vi "OculusRift INTERFACE VI.vi"() -> ()   [LabVIEW 2014]
uses:
  <vilib>/Platform/TimedLoop/XDataNode/timing_clust.ctl
  <vilib>/Platform/TimedLoop/XDataNode/nitl_modes.ctl
  <vilib>/Platform/TimedLoop/XDataNode/wakeup.ctl
  <vilib>/Platform/TimedLoop/XDataNode/XDataNode.xnode
  <vilib>/Platform/TimedLoop/XDataNode/XDNodeRunTimeDep.lvlib
panel:
  in  "LOOP CS":i64=200
  in  "LOOP OR":i64
  in  "service name":string="localhost"
  in  "port":u16=6340
  out "error out":errorcluster
  out "data out":string
  in  "error in (no error) 2":errorcluster
  in  "error in (no error)":errorcluster
  in  "OR Port":u16=52717
  in  "Oculus Rift Adress":string="localhost"
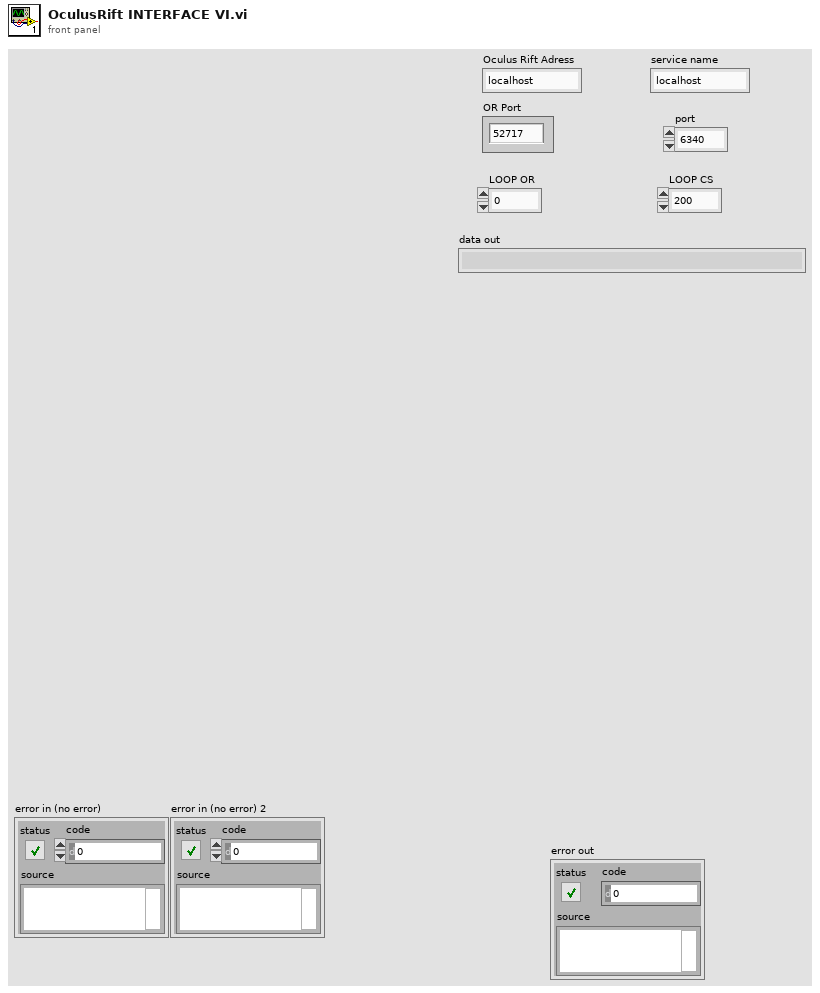
[diagram p1: front panel]
types:
  T1 = typedef "XDNodeRunTimeDep.lvlib/timing_clust.ctl" = cluster{"Expected End [f-1]":u64, "Actual End [f-1]":u64, "Finished Late? [f-1]":bool, "Expected End [i-1]":u64, "Actual End [i-1]":u64, "Finished Late? [i-1]":bool, "Expected Start [i]":u64, "Actual Start [i]":u64, "Expected Start [f]":u64, "Actual Start [f]":u64, "Source Name":string, "Structure Name":string, "Period":i64, "Deadline":i64, "Offset":i64, "Start":i64, "Priority":i32, "Timeout":i32, "Mode":T2, "Wakeup Reason":T3, "Error":errorcluster, "Source Type":string, "Secondary Source Type":string, "Global End Time":u64, "Global Start Time":u64, "Frame Duration":u64, "Iteration Duration":u64, "Assigned CPU":i32, "I/O Scan Engine Mode":u32}
  T2 = typedef "XDNodeRunTimeDep.lvlib/nitl_modes.ctl" = enum32{"No Change", "Process missed periods, maintain original phase", "Discard missed periods, maintain original phase", "Process missed periods, ignore original phase", "Discard missed periods, ignore original phase"}
  T3 = typedef "XDNodeRunTimeDep.lvlib/wakeup.ctl" = enum32{"Normal", "Aborted", "Asynchronous wakeup", "Timing source error", "Timed loop error", "Timeout"}
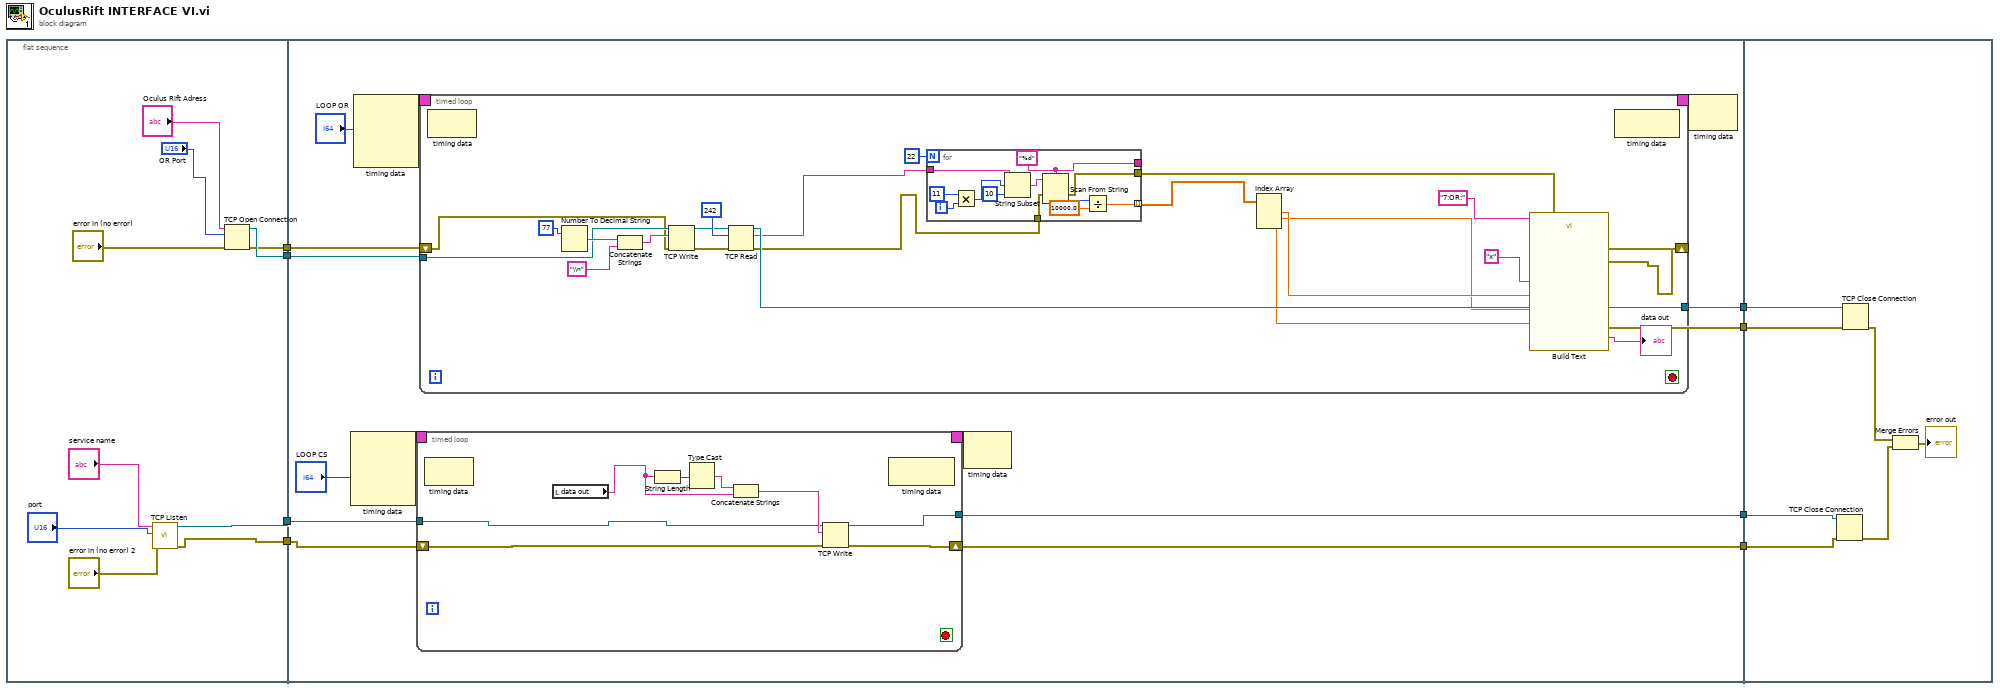
[diagram p0: block diagram]
diagram:
  n1 = flat-sequence {
    tunnel: [w18] -> w8
    tunnel: [w17] -> w7
    tunnel: [w14] -> w6
    tunnel: [w15] -> w1
    tunnel: w8 -> [w30]
    tunnel: w7 -> [w29]
    tunnel: w6 -> [w28]
    tunnel: [w27] -> w5
    tunnel: [w26] -> w4
    tunnel: [w25] -> w3
    tunnel: [w24] -> w2
    tunnel: w1 -> [w22]
    tunnel: w5 -> [w92]
    tunnel: w4 -> [w91]
    tunnel: w3 -> [w90]
    tunnel: w2 -> [w89]
    frame #0 {
      n2 = call <vilib>:"TCP Listen.vi"("error in (no error)"="error in (no error) 2", "port"="port", "service name"="service name") -> ("error out"=w14:errorcluster, "connection ID"=w15:refnum<k5>)  [unwired: 4 in, 3 out]
      n3 = TCP Open Connection(address="Oculus Rift Adress", remote port or service name="OR Port", error in (no error)="error in (no error)") -> (connection ID=w18:refnum<k5>, error out=w17:errorcluster)  [unwired: 2 in]
    }
    frame #1 {
      n4 = node-c288("LOOP CS") -> (w32:T1)  [unwired: 3 in]
      n5 = node-c288("LOOP OR") -> (w21:T1)  [unwired: 3 in]
      n6 = timed-loop {
        timing: w32 -> [_]
        timing-out: [_] -> w31
        shift-right: [w79] -> w26
        shift-left: w28 -> [w73]
        tunnel: [w78] -> w27
        tunnel: w22 -> [w74]
        stop <- _ stop-if-true
        n7 = node-c288() -> ()  [unwired: 1 in, 1 out]
        n8 = local read "data out"() -> (w72:string)
        n9 = String Length(string=w72) -> (length=w77:i32)
        n10 = Type Cast(x=w77) -> (*(type *) &x=w76:string)  [unwired: 1 in]
        n11 = Concatenate Strings(w76, w72) -> (w75:string)
        n12 = TCP Write(connection ID=w74, data in=w75, error in (no error)=w73) -> (connection ID out=w78:refnum<k5>, error out=w79:errorcluster)  [unwired: 1 in, 1 out]
        n13 = node-c288() -> ()  [unwired: 1 in, 1 out]
      }
      n14 = timed-loop {
        timing: w21 -> [_]
        timing-out: [_] -> w20
        tunnel: w30 -> [w46]
        shift-right: [w34] -> w24
        shift-left: w29 -> [w45]
        tunnel: [w44] -> w25
        stop <- _ stop-if-true
        n15 = node-c288() -> ()  [unwired: 1 in, 1 out]
        n16 = Number To Decimal String(number=77) -> (decimal integer string=w49:string)  [unwired: 1 in]
        n17 = Concatenate Strings(w49, "\\n" ("string")) -> (w47:string)
        n18 = TCP Write(connection ID=w46, data in=w47, error in (no error)=w45) -> (connection ID out=w52:refnum<k5>, error out=w51:errorcluster)  [unwired: 1 in, 1 out]
        n19 = TCP Read(connection ID=w52, bytes to read=242, error in (no error)=w51) -> (connection ID out=w44:refnum<k5>, data out=w37:string, error out=w35:errorcluster)  [unwired: 2 in]
        n20 = for {
          N: 22 -> [_]
          tunnel: w37 -> [w65]
          tunnel: [w58] -> w41 mode=indexing
          tunnel: w35 -> [w56]
          tunnel: [w55] -> w34
          tunnel: [w54] -> _
          i -> [w63]
          w54 = "%d" ("format string")
          n21 = Multiply(x=11, y=w63) -> (x*y=w61:i32)
          n22 = String Subset(string=w65, offset (0)=w61, length (rest)=10 ("length (rest)")) -> (substring=w60:string)
          n23 = Scan From String(format string=w54, input string=w60, error in=w56) -> (error out=w55:errorcluster, output 1=w57:i32)  [unwired: 2 in, 2 out]
          n24 = Divide(x=w57, y=10000.0) -> (x/y=w58:dbl)
        }
        n25 = Index Array(array=w41) -> (element #1=w40:dbl, element #2=w39:dbl, element #3=w38:dbl)  [unwired: 3 in]
        n26 = call "Build Text"("Beginning Text"="7:OR:", "val3"=w38, "ORStatus"="x", "val1"=w40, "val2"=w39) -> ("Result"=→"data out":string)  [unwired: 9 in, 1 out]
        n27 = node-c288() -> ()  [unwired: 1 in, 1 out]
      }
      n28 = node-c288(w31) -> ()  [unwired: 1 out]
      n29 = node-c288(w20) -> ()  [unwired: 1 out]
    }
    frame #2 {
      n30 = TCP Close Connection(connection ID=w92, error in (no error)=w91) -> (error out=w87:errorcluster)  [unwired: 1 in, 1 out]
      n31 = TCP Close Connection(connection ID=w90, error in (no error)=w89) -> (error out=w88:errorcluster)  [unwired: 1 in, 1 out]
      n32 = Merge Errors(w88, w87) -> (→"error out":errorcluster)
    }
  }
